vi "Nom fichier_SD.vi"() -> (0 "nom":string="081023_16:37:04")   [LabVIEW 2015]
panel:
  out "chaîne d'heure":string
  out "date à l'allemande":string="081023"
  out "date":string="23/10/2008"
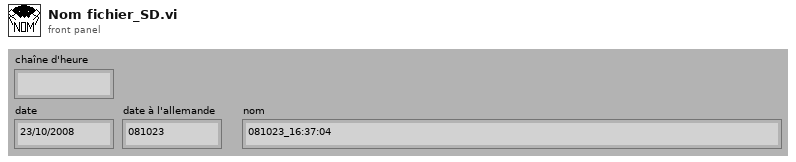
[diagram p1: front panel]
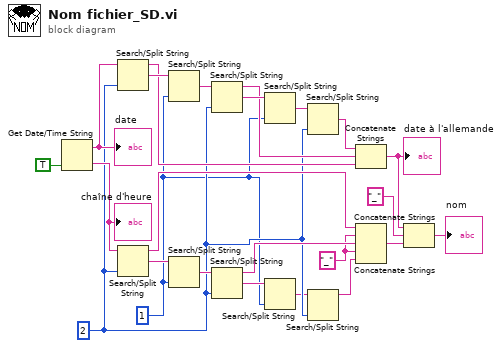
[diagram p0: block diagram]
diagram:
  w6 = "_" ("chaîne")
  w2 = 1 ("offset (0)")
  w4 = 2 ("offset (0)")
  n1 = Get Date/Time String(want seconds? (F)=TRUE ("secondes ? (F)")) -> (date string=w24:string, time string=w11:string)  [unwired: 2 in]
  "date" <- w24
  "chaîne d'heure" <- w11
  n2 = Search/Split String(string=w24, offset (0)=w4) -> (substring before match=w18:string, match + rest of string=w23:string)  [unwired: 1 in, 1 out]
  n3 = Search/Split String(string=w11, offset (0)=w4) -> (substring before match=w10:string, match + rest of string=w9:string)  [unwired: 1 in, 1 out]
  n4 = Search/Split String(string=w23, offset (0)=w2) -> (match + rest of string=w22:string)  [unwired: 1 in, 2 out]
  n5 = Search/Split String(string=w9, offset (0)=w2) -> (match + rest of string=w8:string)  [unwired: 1 in, 2 out]
  n6 = Search/Split String(string=w22, offset (0)=w4) -> (substring before match=w19:string, match + rest of string=w21:string)  [unwired: 1 in, 1 out]
  n7 = Search/Split String(string=w8, offset (0)=w4) -> (substring before match=w7:string, match + rest of string=w5:string)  [unwired: 1 in, 1 out]
  n8 = Search/Split String(string=w21, offset (0)=w2) -> (match + rest of string=w20:string)  [unwired: 1 in, 2 out]
  n9 = Search/Split String(string=w5, offset (0)=w2) -> (match + rest of string=w3:string)  [unwired: 1 in, 2 out]
  n10 = Search/Split String(string=w20, offset (0)=w4) -> (match + rest of string=w17:string)  [unwired: 1 in, 2 out]
  n11 = Search/Split String(string=w3, offset (0)=w4) -> (substring before match=w1:string)  [unwired: 1 in, 2 out]
  n12 = Concatenate Strings(w17, w19, w18) -> (w14:string)
  "date à l'allemande" <- w14
  n13 = Concatenate Strings(w10, w6, w7, w6, w1) -> (w12:string)
  n14 = Concatenate Strings(w14, "_" ("chaîne"), w12) -> (→"nom":string)
